vi "Configure_PSG_ Frequency_Power_final.vi"(0 "RF Output (T:On)":bool=TRUE, 1 "Attenuator Auto Mode (T:Enable)":bool=TRUE, 2 "Power [dBm]":dbl=-130.0, 3 "Frequency [GHz]":dbl=1.0, 4 "VISA resource name":refnum<visa-resource-name>) -> ()   [LabVIEW 2011]
doc: "This example shows how to configure the frequency and power of the output signal."
uses:
  <vilib>/Utility/error.llb/DialogType.ctl
  <instrlib>/Agilent PSG MXG Series/Agilent PSG MXG Series.lvlib
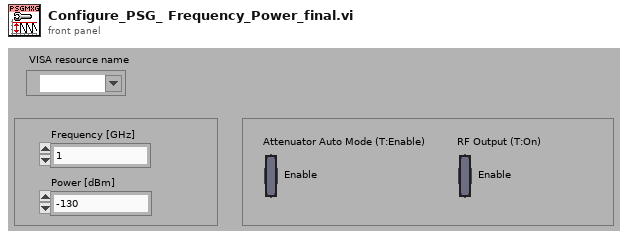
[diagram p1: front panel]
types:
  T1 = typedef "DialogType.ctl" = u16
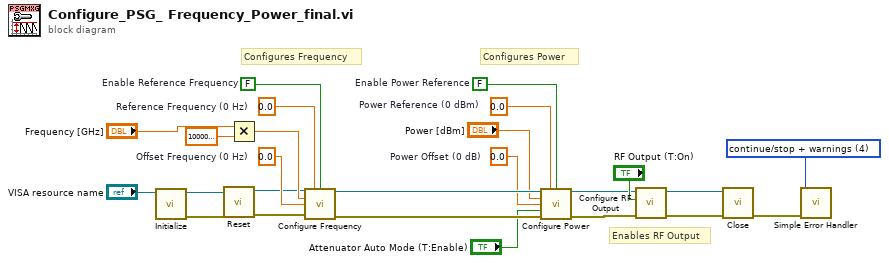
[diagram p0: block diagram]
diagram:
  w1 = T1 4 items=["no dialog", "OK message", "continue or stop message", "OK message + warnings", "continue/stop + warnings"] ("type of dialog (OK msg:1)")
  w16 = 0.0  # Offset Frequency (0 Hz)
  w17 = 0.0  # Reference Frequency (0 Hz)
  w14 = 0.0  # Power Reference (0 dBm)
  w13 = 0.0  # Power Offset (0 dB)
  w15 = FALSE  # Enable Power Reference
  w18 = FALSE  # Enable Reference Frequency
  # "Enables RF Output"
  # "Configures Power"
  # "Configures Frequency"
  n1 = call <instrlib>:"Initialize.vi"("VISA resource name"="VISA resource name") -> ("error out"=w3:errorcluster, "VISA resource name out"=w5:refnum<visa-resource-name>)  [unwired: 9 in]
  n2 = call <instrlib>:"Reset.vi"("error in (no error)"=w3, "VISA resource name"=w5) -> ("error out"=w2:errorcluster, "VISA resource name out"=w4:refnum<visa-resource-name>)  [unwired: 8 in]
  n3 = Multiply(x="Frequency [GHz]", y=1000000000.0) -> (x*y=w6:dbl)
  n4 = call <instrlib>:"Configure Frequency.vi"("VISA resource name"=w4, "Reference Frequency (0 Hz)"=w17, "Enable Reference Frequency (F:Disable)"=w18, "Frequency (100 kHz)"=w6, "Offset Frequency (0 Hz)"=w16, "error in (no error)"=w2) -> ("VISA resource name out"=w25:refnum<visa-resource-name>, "error out"=w24:errorcluster)  [unwired: 8 in]
  n5 = call <instrlib>:"Configure Power.vi"("VISA resource name"=w25, "Power Reference (0 dBm)"=w14, "Enable Power Reference (F:Disable)"=w15, "Power (-130 dBm)"="Power [dBm]", "Power Offset (0 dB)"=w13, "Attenuator Auto Mode (T:Enable)"="Attenuator Auto Mode (T:Enable)", "error in (no error)"=w24) -> ("VISA resource name out"=w10:refnum<visa-resource-name>, "error out"=w9:errorcluster)  [unwired: 7 in]
  n6 = call <instrlib>:"Configure RF Output.vi"("error in (no error)"=w9, "Enable RF Output (F:Disable)"="RF Output (T:On)", "VISA resource name"=w10) -> ("error out"=w21:errorcluster, "VISA resource name out"=w22:refnum<visa-resource-name>)  [unwired: 7 in]
  n7 = call <instrlib>:"Close.vi"("error in (no error)"=w21, "VISA resource name"=w22) -> ("error out"=w23:errorcluster)  [unwired: 9 in]
  n8 = call <vilib>:"Simple Error Handler.vi"("type of dialog (OK msg:1)"=w1, "error in (no error)"=w23) -> ()  [unwired: 3 in, 5 out]
